vi "pp3_DAQclear.vi"(8 "error in (no error)":errorcluster, 11 "Daq config in":T1={"Sound AO"="Dev6/ao0", "Shock intesity AO"="Dev6/ao1", "Code_LED DO"="Dev6/port1:2", "Switch DI"="Dev6/port1/line0", "Webcam"="cam9", "Sound AO task"="", "Sound card task"=0, "Shock intensity AO task"="", "Code_LED DO task"="", "Switch DI task"="", "AO <=> Sound card"=FALSE, "Sound card"=0, "sample rate"=100000.0, "Variable shock"=TRUE, "Webcam on"=FALSE, "Waveform memo"={"t0"=timestamp(0 s since 1904-01-01), "dt"=1.0, "Y"=[]}, "First time"=FALSE, "Tone trigger"="", "Master-9 DO"="Dev6/port0/line5:7", "Master-9 DO task"=""} {"sample rate" min=8000.0; "Sound card task" format="%.0x"}) -> (0 "error out":errorcluster, 3 "Daq config out":T1={"Sound AO"="Dev6/ao0", "Shock intesity AO"="Dev6/ao1", "Code_LED DO"="Dev6/port1:2", "Switch DI"="Dev6/port1/line0", "Webcam"="cam9", "Sound AO task"="", "Sound card task"=0, "Shock intensity AO task"="", "Code_LED DO task"="", "Switch DI task"="", "AO <=> Sound card"=FALSE, "Sound card"=0, "sample rate"=100000.0, "Variable shock"=TRUE, "Webcam on"=FALSE, "Waveform memo"={"t0"=timestamp(0 s since 1904-01-01), "dt"=1.0, "Y"=[]}, "First time"=FALSE, "Tone trigger"="", "Master-9 DO"="Dev6/port0/line5:7", "Master-9 DO task"=""} {"sample rate" min=8000.0; "Sound card task" format="%.0x"})   [LabVIEW 2013]
uses:
  pp3b_CTL_DaqConfig.ctl
  <vilib>/userdefined/High Color/IMAQdx.ctl
  <vilib>/sound2/lvsound2.llb/Sound Output Task ID.ctl
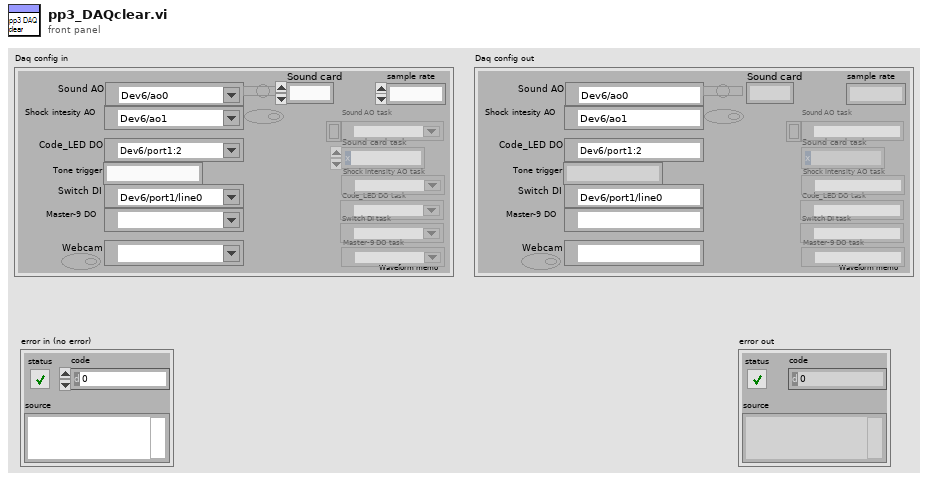
[diagram p1: front panel]
types:
  T1 = typedef "pp3b_CTL_DaqConfig.ctl" = cluster{"Sound AO":tag, "Shock intesity AO":tag, "Code_LED DO":tag, "Switch DI":tag, "Webcam":T2, "Sound AO task":refnum<k21>, "Sound card task":T3, "Shock intensity AO task":refnum<k21>, "Code_LED DO task":refnum<k21>, "Switch DI task":refnum<k21>, "AO <=> Sound card":bool, "Sound card":u32, "sample rate":dbl, "Variable shock":bool, "Webcam on":bool, "Waveform memo":waveform(dbl), "First time":bool, "Tone trigger":string, "Master-9 DO":tag, "Master-9 DO task":refnum<k21>}
  T2 = typedef "IMAQdx.ctl" = refnum<k21>
  T3 = typedef "Sound Output Task ID.ctl" = u32
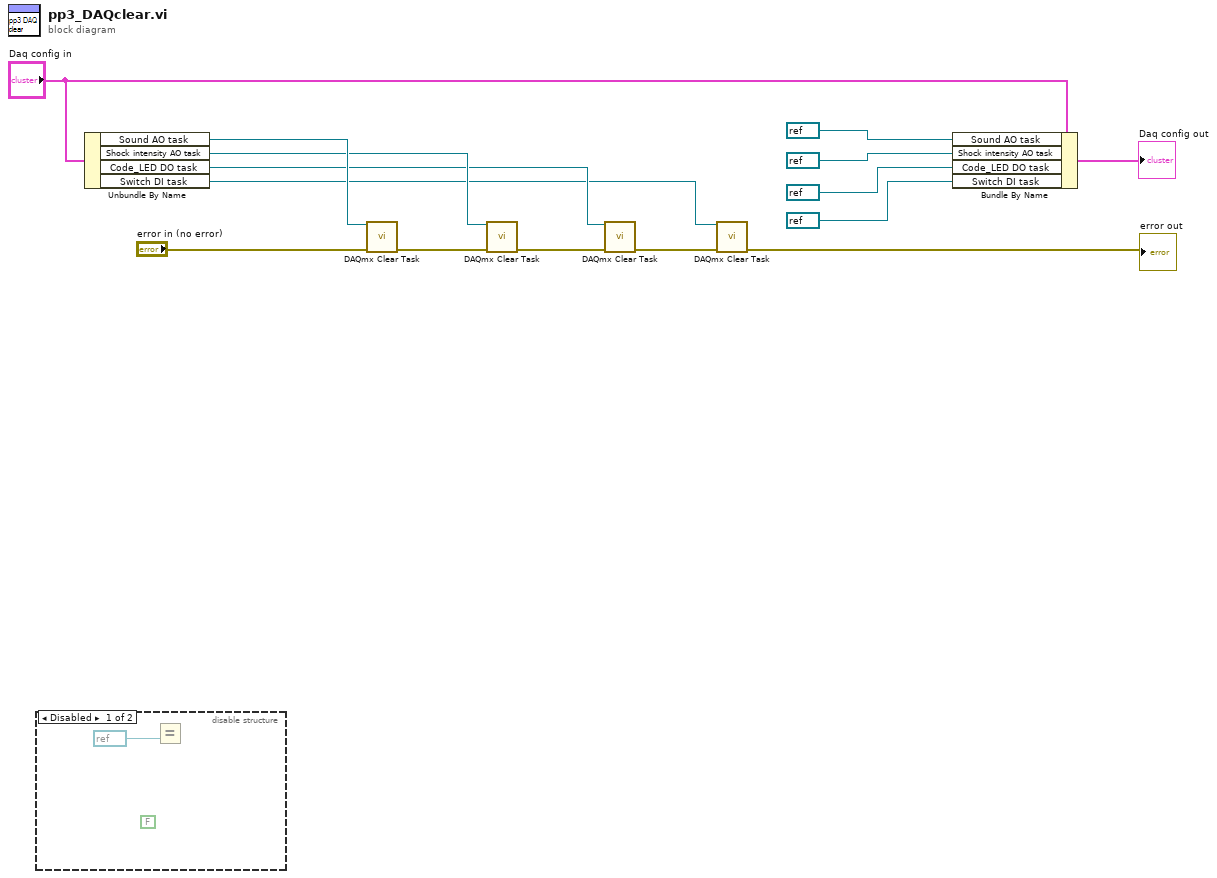
[diagram p0: block diagram]
diagram:
  n1 = disable-structure shown="Disabled" {
    frame Disabled {
      (unwired) FALSE
      n2 = Equal?(y=refnum<k21> refnum) -> ()  [unwired: 1 in, 1 out]
    }
    frame Enabled {
    }
  }
  n3 = Unbundle By Name("Daq config in") -> ("Sound AO task"=w12:refnum<k21>, "Shock intensity AO task"=w7:refnum<k21>, "Code_LED DO task"=w2:refnum<k21>, "Switch DI task"=w1:refnum<k21>)
  n4 = call <vilib>:"DAQmx Clear Task.vi"("task in"=w12, "error in"="error in (no error)") -> ("error out"=w6:errorcluster)  [unwired: 13 in]
  n5 = call <vilib>:"DAQmx Clear Task.vi"("task in"=w7, "error in"=w6) -> ("error out"=w5:errorcluster)  [unwired: 13 in]
  n6 = call <vilib>:"DAQmx Clear Task.vi"("task in"=w2, "error in"=w5) -> ("error out"=w4:errorcluster)  [unwired: 13 in]
  n7 = call <vilib>:"DAQmx Clear Task.vi"("task in"=w1, "error in"=w4) -> ("error out"=→"error out":errorcluster)  [unwired: 13 in]
  n8 = Bundle By Name(cluster="Daq config in", "Sound AO task"=refnum<k21> refnum ("NULL"), "Shock intensity AO task"=refnum<k21> refnum ("NULL"), "Code_LED DO task"=refnum<k21> refnum ("NULL"), "Switch DI task"=refnum<k21> refnum ("NULL")) -> (→"Daq config out":T1)
